vi "Draw PlotImageFront.vi"(8 "error in (no error)":errorcluster, 9 "Coords":T1, 10 "Refs":T12, 11 "Loop data in":T2={"TitleCollapse"=refnum, "MouseDownState"=enum."Idle", "RightClickCache"={"Mod"={"Ctrl"=FALSE, "Shift"=FALSE}, "CoordsStart"={"Horizontal"=0, "Vertical"=0}, "CoordsEnd"={"Horizontal"=0, "Vertical"=0}, "PlotAreaBounds"={"Left"=10, "Top"=10, "Right"=0, "Bottom"=0}, "slice"=[]}, "ZoomCache"={"SuppressedPlots"=[], "LeftAxis"={"NeedsRevert?"=FALSE, "Scale Fit"=0, "Range"={"Minimum"=0.0, "Maximum"=0.0, "Increment"=0.0, "Minor Increment"=0.0, "Start"=0.0}}, "RightAxis"={"NeedsRevert?"=FALSE, "Scale Fit"=0, "Range"={"Minimum"=0.0, "Maximum"=0.0, "Increment"=0.0, "Minor Increment"=0.0, "Start"=0.0}}, "Mod"={"Shift"=FALSE}}, "UpdateTime"=0.0, "keyboard"=refnum, "visible?"=FALSE}) -> (0 "error out":errorcluster, 3 "Loop data out":T2={"TitleCollapse"=refnum, "MouseDownState"=enum."Idle", "RightClickCache"={"Mod"={"Ctrl"=FALSE, "Shift"=FALSE}, "CoordsStart"={"Horizontal"=0, "Vertical"=0}, "CoordsEnd"={"Horizontal"=0, "Vertical"=0}, "PlotAreaBounds"={"Left"=10, "Top"=10, "Right"=0, "Bottom"=0}, "slice"=[]}, "ZoomCache"={"SuppressedPlots"=[], "LeftAxis"={"NeedsRevert?"=FALSE, "Scale Fit"=0, "Range"={"Minimum"=0.0, "Maximum"=0.0, "Increment"=0.0, "Minor Increment"=0.0, "Start"=0.0}}, "RightAxis"={"NeedsRevert?"=FALSE, "Scale Fit"=0, "Range"={"Minimum"=0.0, "Maximum"=0.0, "Increment"=0.0, "Minor Increment"=0.0, "Start"=0.0}}, "Mod"={"Shift"=FALSE}}, "UpdateTime"=0.0, "keyboard"=refnum, "visible?"=FALSE})   [LabVIEW 2021, in "RocketPlot.lvlib"]
uses:
  RocketPlot.lvlib
  TypeDefs/Plot UI references.ctl
  Classes/RocketPlotHandle/RocketPlotHandle.lvclass
  <userlib>/bjustice/TipStripOOPanel/Classes/TipPanelHandle/TipPanelHandle.lvclass
  TypeDefs/Plot top row.ctl
  TypeDefs/plot while loop data.ctl
  CollapsePanel/CollapsePanel.lvclass
  TypeDefs/MouseDownState.ctl
  TypeDefs/RightClickCache.ctl
  TypeDefs/RightClickCache PlatMod.ctl
  <vilib>/Utility/miscctls.llb/LVPoint32TypeDef.ctl
  <vilib>/Utility/miscctls.llb/LVRectTypeDef.ctl
  TypeDefs/Slice average.ctl
  TypeDefs/ZoomCache.ctl
  TypeDefs/RangeCache.ctl
  <vilib>/Utility/miscctls.llb/LVRangeTypeDef.ctl
  TypeDefs/ZoomCache PlatMod.ctl
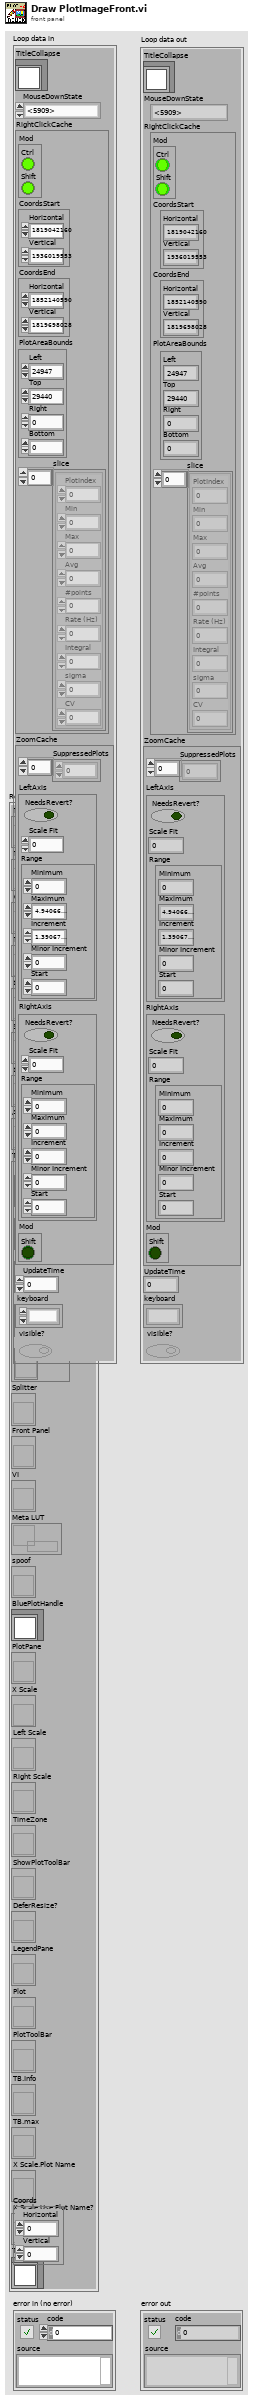
[diagram p1: front panel]
types:
  T1 = typedef "LVPoint32TypeDef.ctl" = cluster{"Horizontal":i32, "Vertical":i32}
  T2 = typedef "RocketPlot.lvlib/plot while loop data.ctl" = cluster{"TitleCollapse":refnum<class "CollapsePanel.lvclass">, "MouseDownState":T3, "RightClickCache":T4, "ZoomCache":T8, "UpdateTime":dbl, "keyboard":refnum<k1>, "visible?":bool}
  T3 = typedef "RocketPlot.lvlib/MouseDownState.ctl" = enum16{"Idle", "Pan", "Zoom", "Zoom-Post", "RightClick"}
  T4 = typedef "RocketPlot.lvlib/RightClickCache.ctl" = cluster{"Mod":T5, "CoordsStart":T1, "CoordsEnd":T1, "PlotAreaBounds":T6, "slice":T7[]}
  T5 = typedef "RocketPlot.lvlib/RightClickCache PlatMod.ctl" = cluster{"Ctrl":bool, "Shift":bool}
  T6 = typedef "LVRectTypeDef.ctl" = cluster{"Left":i16, "Top":i16, "Right":i16, "Bottom":i16}
  T7 = typedef "RocketPlot.lvlib/Slice average.ctl" = cluster{"PlotIndex":i32, "Min":dbl, "Max":dbl, "Avg":dbl, "#points":u32, "Rate (Hz)":dbl, "Integral":dbl, "sigma":dbl, "CV":dbl}
  T8 = typedef "RocketPlot.lvlib/ZoomCache.ctl" = cluster{"SuppressedPlots":i32[], "LeftAxis":T9, "RightAxis":T9, "Mod":T11}
  T9 = typedef "RocketPlot.lvlib/RangeCache.ctl" = cluster{"NeedsRevert?":bool, "Scale Fit":u8, "Range":T10}
  T10 = typedef "LVRangeTypeDef.ctl" = cluster{"Minimum":dbl, "Maximum":dbl, "Increment":dbl, "Minor Increment":dbl, "Start":dbl}
  T11 = typedef "RocketPlot.lvlib/ZoomCache PlatMod.ctl" = cluster{"Shift":bool}
  T12 = typedef "RocketPlot.lvlib/Plot UI references.ctl" = cluster{"Title":refnum<vi>, "Title?":refnum<vi>, "Visible sidebar?":refnum<vi>, "Time to Plot":refnum<vi>, "top array":refnum<vi>, "Scrollbar":refnum<vi>, "tab ref":refnum<vi>, "Add row":refnum<vi>, "TopArray":cluster{"PID":refnum<vi>, "Numeric color":refnum<vi>, "Flat":refnum<vi>, "PID color":refnum<vi>, "Data":refnum<vi>}, "Splitter":refnum<vi>, "Front Panel":refnum<vi>, "VI":refnum<vi>, "Meta LUT":refnum<data-value>, "spoof":refnum<vi>, "BluePlotHandle":refnum<class "RocketPlotHandle.lvclass">, "PlotPane":refnum<vi>, "X Scale":refnum<vi>, "Left Scale":refnum<vi>, "Right Scale":refnum<vi>, "TimeZone":refnum<vi>, "ShowPlotToolBar":refnum<vi>, "DeferResize?":refnum<vi>, "LegendPane":refnum<vi>, "Plot":refnum<vi>, "PlotToolBar":refnum<vi>, "TB.Info":refnum<vi>, "TB.max":refnum<vi>, "X Scale.Plot Name":refnum<vi>, "X Scale.Use Plot Name?":refnum<vi>, "TipPanel":refnum<class "TipPanelHandle.lvclass">}
  T13 = typedef "RocketPlot.lvlib/RightClickType.ctl" = enum16{"Idle", "Delta", "SliceAvg", "Identify"}
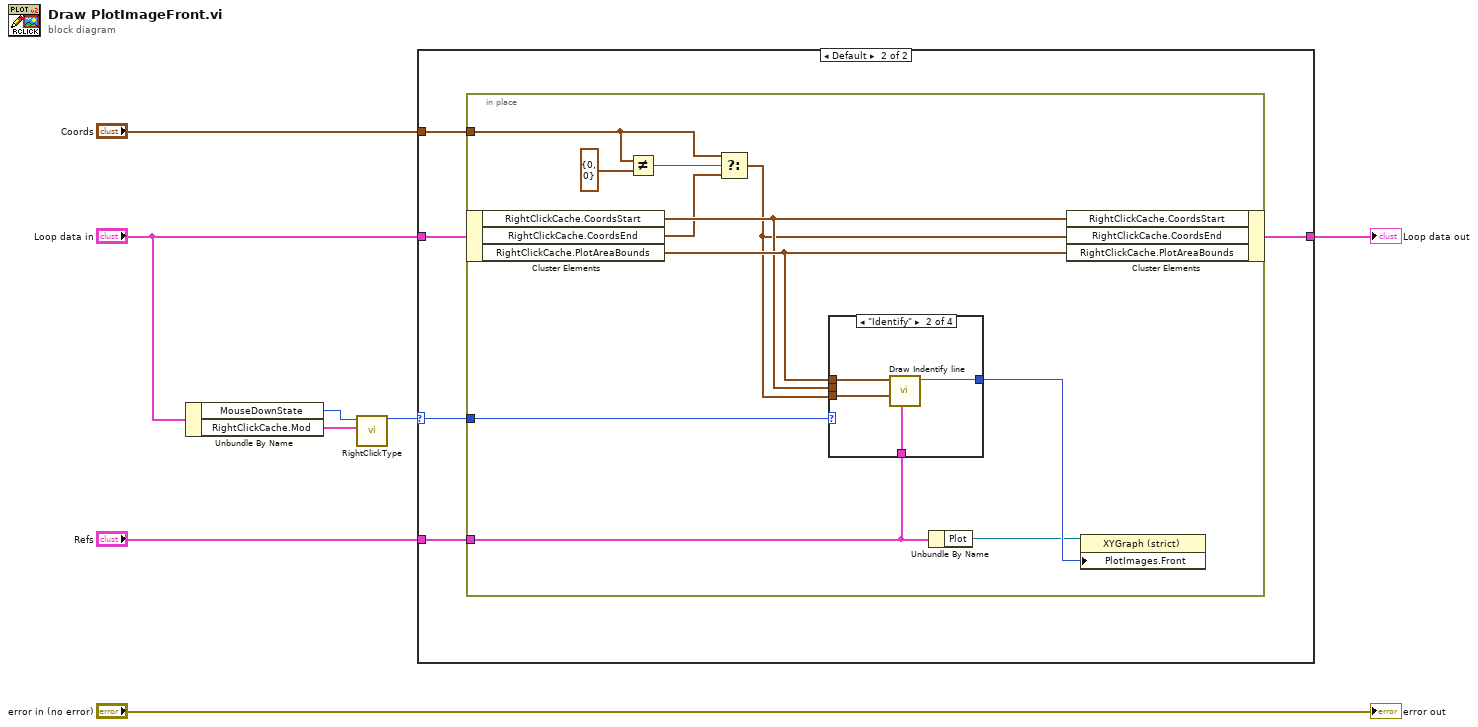
[diagram p0: block diagram]
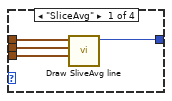
[diagram p3: hidden frame]
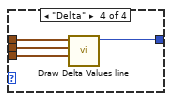
[diagram p5: hidden frame]
diagram:
  n1 = Unbundle By Name("Loop data in") -> ("MouseDownState"=w3:T3, "RightClickCache.Mod"=w4:T5)
  n2 = call "RightClickType.vi"("Mod"=w4, "MouseDownState"=w3) -> ("RightClickType"=w1:T13)  [unwired: 9 in]
  n3 = case shown="Default" w1 {
    selector: w1 -> [_ w10]
    tunnel: "Coords" -> [_ w14]
    tunnel: [w9 w13] -> w6
    tunnel: "Refs" -> [_ w12]
    tunnel: "Loop data in" -> [w9 w11]
    frame "Idle" {
    }
    frame Default {
      n4 = in-place {
        in-place-border: w14 -> [w17]
        in-place-border: w12 -> [w21]
        in-place-border: w10 -> [w20]
        n5 = in-place-cluster #1(w11) -> ("RightClickCache.CoordsStart"=w24:T1, "RightClickCache.CoordsEnd"=w16:T1, "RightClickCache.PlotAreaBounds"=w25:T6)
        n6 = Not Equal?(x=w17, y=T1 {"Horizontal"=0, "Vertical"=0} ("Coords")) -> (x != y?=w18:bool)
        n7 = Select(t=w17, s=w18, f=w16) -> (s? t:f=w15:T1)
        n8 = case shown="\"Identify\"" w20 {
          tunnel: w25 -> [w29 w33 _ w37]
          tunnel: w15 -> [w27 w32 _ w36]
          tunnel: w24 -> [w28 _ _ w35]
          tunnel: [w26 w31 _ w34] -> w23
          tunnel: w21 -> [_ w30 _ _]
          frame "SliceAvg" {
            n9 = call "Draw SliveAvg line.vi"("Coords-end"=w27, "Coords-start"=w28, "PlotAreaBounds"=w29) -> ("picture"=w26:picture)  [unwired: 7 in, 1 out]
          }
          frame "Identify" {
            n10 = call "Draw Indentify line.vi"("Refs"=w30, "Coords-end"=w32, "PlotAreaBounds"=w33) -> ("picture"=w31:picture)  [unwired: 7 in, 1 out]
          }
          frame "Idle" {
          }
          frame "Delta" {
            n11 = call "Draw Delta Values line.vi"("Coords-end"=w36, "Coords-start"=w35, "PlotAreaBounds"=w37) -> ("picture"=w34:picture)  [unwired: 7 in, 1 out]
          }
        }
        n12 = Unbundle By Name(w21) -> ("Plot"=w22:refnum<vi>)
        n13 = in-place-cluster #1("RightClickCache.CoordsStart"=w24, "RightClickCache.CoordsEnd"=w15, "RightClickCache.PlotAreaBounds"=w25) -> (w13:T2)
        n14 = property class="XYGraph (strict)"(reference=w22, "PlotImages.Front"=w23) -> ()  [unwired: 1 in, 2 out]
      }
    }
  }
  "Loop data out" <- w6
  "error out" <- "error in (no error)"
